vi "1_SimpleDemo_MHHisto.vi"() -> ()   [LabVIEW 2020]
uses:
  _lib/PQ/MultiHarp/MH_RefSource.ctl
  _lib/PQ/MultiHarp/MH_MeasMode.ctl
  <vilib>/Utility/error.llb/Error Cluster From Error Code.vi
  _lib/PQ/MultiHarp/MH_LibVersion_global.vi
  _lib/PQ/MultiHarp/mhlib_x86_x64_UIThread.llb/MH_DllPath_global.vi
  <vilib>/ErrorRing/Error Ring.xnode
panel:
  in  "EnableInputDeadTime":bool caption="Enable DeadTime"
  in  "InputDeadTime":i32=1000 caption="DeadTime [ps]" min=800 max=160000 step=1
  in  "Trg.Edge":i32(ring) items=["falling", "rising"]
  in  "Trg.Level":i32=-100 caption="Trg.Level [mV]" min=-1200 max=1200 step=1
  in  "Offset":i32 caption="Offset [ps]" min=-99999 max=99999 step=1
  in  "Enable":bool=TRUE
  in  "EnableSyncDeadTime":bool caption="Enable DeadTime"
  in  "SyncDeadTime":i32=1000 caption="SyncDeadTime [ps]" min=800 max=160000 step=1
  in  "SyncTrg.Edge":i32(ring) items=["falling", "rising"]
  in  "SyncTrg.Level":i32=-100 caption="SyncTrg.Level [mV]" min=-1200 max=1200 step=1
  in  "SyncOffset":i32 caption="SyncOffset [ps]" min=-99999 max=99999 step=1
  in  "SyncDivider":i32(ring)=1 items=["1"=1, "2"=2, "4"=4, "8"=8, "16"=16]
  in  "Binning":i32(ring) caption="Resolution [ps]" items=["5", "10", "20", "40", "80", "160", "320", "640", "1280", "2560", "5120", "10240", "20480", "40960", "81920", "163840", "327680", "655360", "1310720", "2621440", "5242880", "10485760", "20971520", "41943040"]
  in  "HistoLength":i32(ring)=6 caption="Histo Length" items=["1024", "2048", "4096", "8192", "16384", "32768", "65536"]
  in  "Acqu.Time":i32=10000 caption="Acqu.Time [ms]" min=1 max=360000 step=1
  in  "GlobalOffset":i32 caption="GlobalOffset [ns]" min=0 max=100000000 step=1
  in  "OverflowLevel":u32=4294967295 min=1 step=1
  in  "StopOnOverflow":bool=TRUE
  out "HistoGraph":T1(graph)={0.0, "Resolution"=0.08, "Histogram"=array8x65536[524288 elements]}
  out "CountRates":i32[](array[numeric]) caption="Count Rates [cps]"
  out "SyncRate":i32 caption="Sync Rate [cps]"
  in  "stop":bool
  out "error out":errorcluster
  # "All Channels"
  # "Sync"
  # "Acquisition"
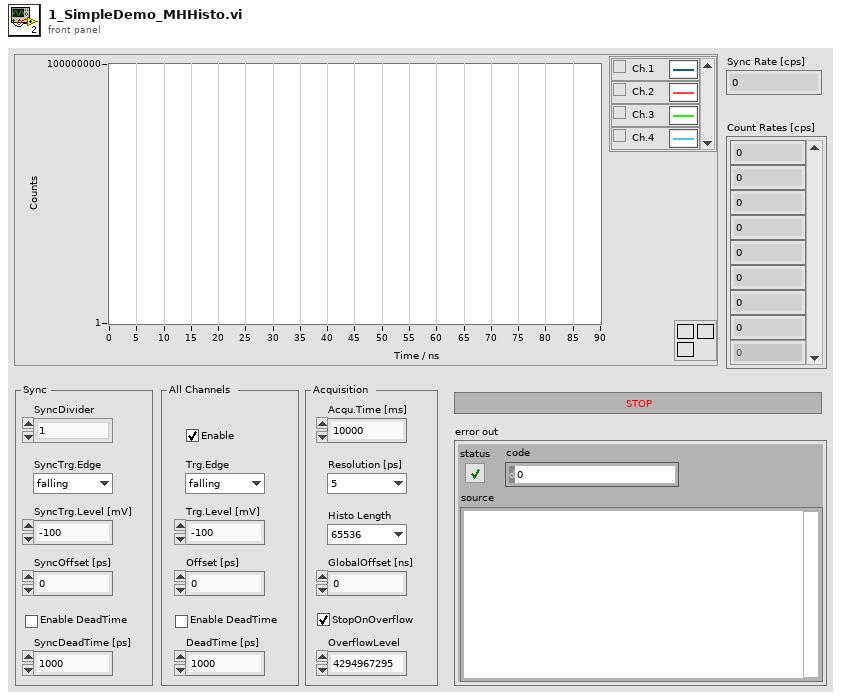
[diagram p1: front panel]
types:
  T1 = cluster{dbl, "Resolution":dbl, "Histogram":u32[][]}
  T2 = typedef "MH_MeasMode.ctl" = i32
  T3 = typedef "MH_RefSource.ctl" = enum16{"INTERNAL", "EXTERNAL_10MHZ", "WR_MASTER_GENERIC", "WR_SLAVE_GENERIC", "WR_GRANDM_GENERIC", "EXTN_GPS_PPS", "EXTN_GPS_PPS_UART", "WR_MASTER_MHARP", "WR_SLAVE_MHARP", "WR_GRANDM_MHARP"}
  T4 = typedef "MH_InitInfo.ctl" = cluster{"Library Version":string, "Serial No.":string, "Model":string, "Partnum":string, "Version":string, "features":i32, "nchannels":i32, "Base Resolution":dbl, "Bin Steps":i32}
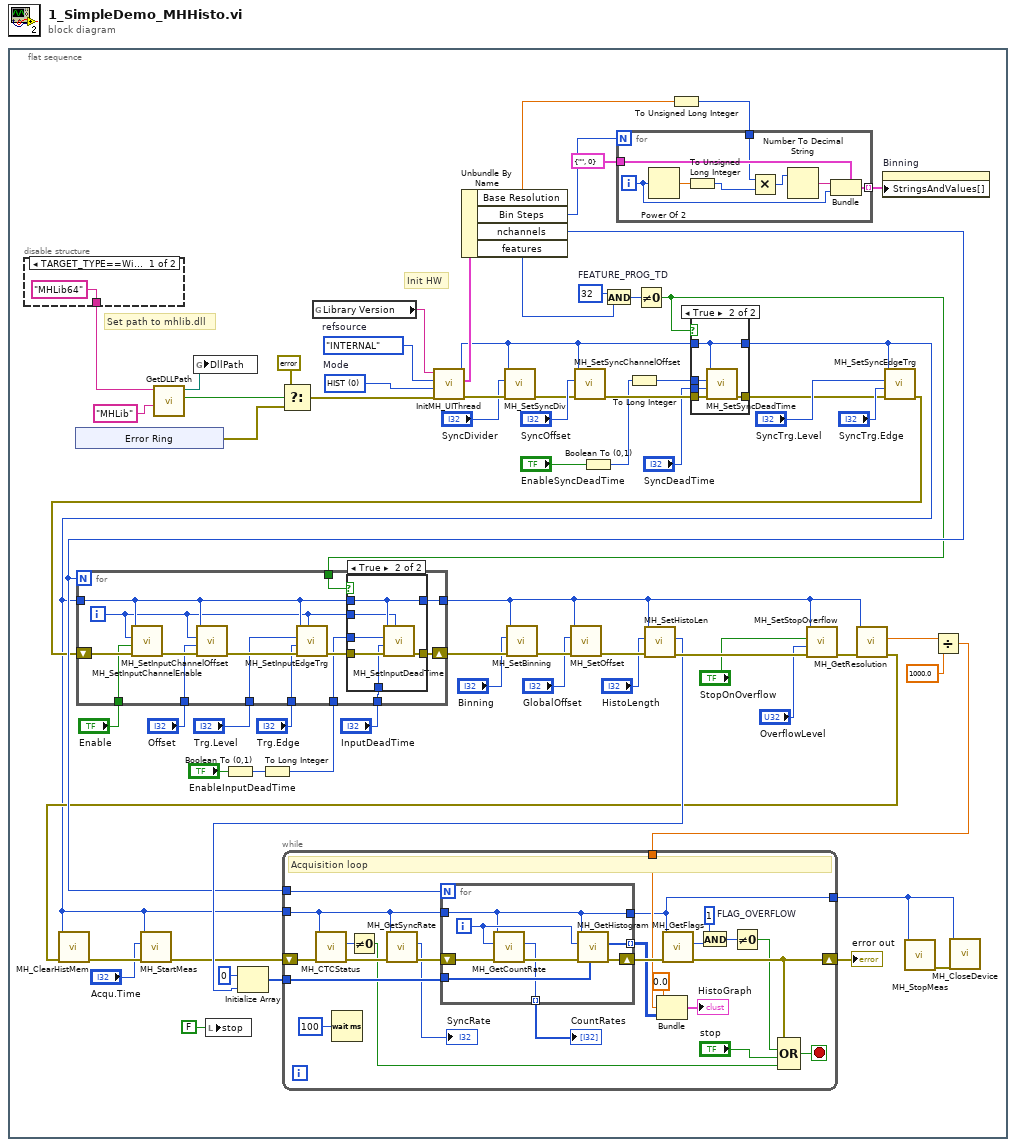
[diagram p0: block diagram]
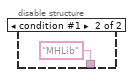
[diagram p3: hidden frame]
diagram:
  n1 = flat-sequence {
    frame #0 {
      w12 = 32  # FEATURE_PROG_TD
      w23 = T2 0 items=["HIST"=0, "T2"=2, "T3"=3]  # Mode
      w69 = MH_RefSource."INTERNAL"  # refsource
      # "Init HW"
      # "Set path to mhlib.dll"
      n2 = disable-structure shown="TARGET_TYPE==Windows, Default" {
        disable-tunnel: ["MHLib64" ("name or relative path") "MHLib" ("name or relative path")] -> w22
        frame condition #0 (active) {
        }
        frame condition #1 {
        }
      }
      n3 = xnode "Error Ring"() -> ("error out"=w68:errorcluster)
      n4 = call "GetDLLPath.vi"("DllName_32bit"="MHLib" ("name or relative path"), "DllName_64bit"=w22) -> ("file exists?"=w66:bool, "DLLPath"=w65:path)  [unwired: 8 in]
      n5 = global write "MH_DllPath_global.vi" "DllPath"(w65) -> ()
      n6 = local write "stop"(FALSE ("stop")) -> ()
      n7 = Boolean To (0,1)(Boolean="EnableInputDeadTime") -> (0, 1=w8:i16)
      n8 = To Long Integer(number=w8) -> (32bit integer=w7:i32)
      n9 = Select(t=errorcluster {"status"=FALSE, "code"=0, "source"=""} ("error IO"), s=w66, f=w68) -> (s? t:f=w63:errorcluster)
      n10 = global read "MH_LibVersion_global.vi" "Library Version"() -> (w26:string)
      n11 = call "InitMH_UIThread.vi"("error in (no error)"=w63, "Mode"=w23, "refsource"=w69, "Library Version"=w26) -> ("error out"=w58:errorcluster, "Init Info"=w60:T4, "DevIdx"=w19:i32)  [unwired: 5 in]
      n12 = Unbundle By Name(w60) -> ("Base Resolution"=w3:dbl, "Bin Steps"=w4:i32, "nchannels"=w40:i32, "features"=w14:i32)
      n13 = call "MH_SetSyncDiv.vi"("error in (no error)"=w58, "SyncDivider"="SyncDivider", "devidx"=w19) -> ("error out"=w57:errorcluster)  [unwired: 7 in, 1 out]
      n14 = call "MH_SetSyncChannelOffset.vi"("error in (no error)"=w57, "Offset"="SyncOffset", "devidx"=w19) -> ("error out"=w21:errorcluster)  [unwired: 7 in, 1 out]
      n15 = Boolean To (0,1)(Boolean="EnableSyncDeadTime") -> (0, 1=w17:i16)
      n16 = And(x=w12, y=w14) -> (x .and. y?=w13:i32)
      n17 = To Long Integer(number=w17) -> (32bit integer=w16:i32)
      n18 = Not Equal To 0?(x=w13) -> (x != 0?=w6:bool)
      n19 = To Unsigned Long Integer(number=w3) -> (unsigned 32bit integer=w2:u32)
      n20 = for {
        N: w4 -> [_]
        tunnel: cluster{"String":string, "Value":i32} {"String"="", "Value"=0} -> [w77]
        tunnel: [w71] -> w1 mode=indexing
        tunnel: w2 -> [w70]
        i -> [w76]
        n21 = Power Of 2(x=w76) -> (2^x=w75:dbl)
        n22 = To Unsigned Long Integer(number=w75) -> (unsigned 32bit integer=w74:u32)
        n23 = Multiply(x=w70, y=w74) -> (x*y=w73:u32)
        n24 = Number To Decimal String(number=w73) -> (decimal integer string=w72:string)  [unwired: 1 in]
        n25 = Bundle(cluster=w77, "String"=w72, "Value"=w76) -> (w71:cluster{"String":string, "Value":i32})
      }
      n26 = case shown="True" w6 {
        tunnel: w21 -> [w78 w84]
        tunnel: [w78 w83] -> w20
        tunnel: w19 -> [w79 w80]
        tunnel: w16 -> [_ w82]
        tunnel: "SyncDeadTime" -> [_ w81]
        tunnel: [w79 w80] -> w11
        frame False {
        }
        frame True {
          n27 = call "MH_SetSyncDeadTime.vi"("error in (no error)"=w84, "deadtime"=w81, "on"=w82, "devidx"=w80) -> ("error out"=w83:errorcluster)  [unwired: 6 in, 1 out]
        }
      }
      n28 = property on="Binning" class="Ring (strict)"("StringsAndValues[]"=w1) -> ()  [unwired: 2 in, 2 out]
      n29 = call "MH_SetSyncEdgeTrg.vi"("error in (no error)"=w20, "edge"="SyncTrg.Edge", "level"="SyncTrg.Level", "devidx"=w11) -> ("error out"=w39:errorcluster)  [unwired: 6 in, 1 out]
      n30 = for {
        N: w40 -> [_]
        shift-right: [w124] -> w59
        shift-left: w39 -> [w133]
        tunnel: w11 -> [w125]
        tunnel: [w123] -> w34
        tunnel: "Enable" -> [w130]
        tunnel: "Offset" -> [w129]
        tunnel: "Trg.Edge" -> [w128]
        tunnel: "Trg.Level" -> [w127]
        tunnel: "InputDeadTime" -> [w121]
        tunnel: w7 -> [w120]
        tunnel: w6 -> [w119]
        i -> [w122]
        n31 = call "MH_SetInputChannelEnable.vi"("error in (no error)"=w133, "enable"=w130, "channel"=w122, "devidx"=w125) -> ("error out"=w132:errorcluster)  [unwired: 6 in, 1 out]
        n32 = call "MH_SetInputChannelOffset.vi"("error in (no error)"=w132, "Offset"=w129, "channel"=w122, "devidx"=w125) -> ("error out"=w131:errorcluster)  [unwired: 6 in, 1 out]
        n33 = call "MH_SetInputEdgeTrg.vi"("channel"=w122, "error in (no error)"=w131, "edge"=w128, "level"=w127, "devidx"=w125) -> ("error out"=w126:errorcluster)  [unwired: 5 in, 1 out]
        n34 = case shown="True" w119 {
          tunnel: w126 -> [w135 w141]
          tunnel: w125 -> [w134 w139]
          tunnel: [w135 w140] -> w124
          tunnel: [w134 w139] -> w123
          tunnel: w122 -> [_ w138]
          tunnel: w121 -> [_ w137]
          tunnel: w120 -> [_ w136]
          frame False {
          }
          frame True {
            n35 = call "MH_SetInputDeadTime.vi"("channel"=w138, "error in (no error)"=w141, "deadtime"=w137, "on"=w136, "devidx"=w139) -> ("error out"=w140:errorcluster)  [unwired: 5 in, 1 out]
          }
        }
      }
      n36 = call "MH_SetBinning.vi"("error in (no error)"=w59, "Binning"="Binning", "devidx"=w34) -> ("error out"=w55:errorcluster)  [unwired: 7 in, 1 out]
      n37 = call "MH_SetOffset.vi"("error in (no error)"=w55, "Offset"="GlobalOffset", "devidx"=w34) -> ("error out"=w53:errorcluster)  [unwired: 7 in, 1 out]
      n38 = call "MH_SetHistoLen.vi"("error in (no error)"=w53, "lencode"="HistoLength", "devidx"=w34) -> ("error out"=w52:errorcluster, "actuallen"=w45:i32)  [unwired: 6 in, 1 out]
      n39 = Initialize Array(u32 0, w45) -> (w44:u32[])
      n40 = call "MH_SetStopOverflow.vi"("error in (no error)"=w52, "stopcount"="OverflowLevel", "StopOnOverflow"="StopOnOverflow", "devidx"=w34) -> ("error out"=w35:errorcluster)  [unwired: 6 in, 1 out]
      n41 = call "MH_GetResolution.vi"("error in (no error)"=w35, "devidx"=w34) -> ("error out"=w32:errorcluster, "resolution"=w33:dbl)  [unwired: 7 in, 1 out]
      n42 = call "MH_ClearHistMem.vi"("error in (no error)"=w32, "devidx"=w11) -> ("error out"=w49:errorcluster)  [unwired: 8 in, 1 out]
      n43 = call "MH_StartMeas.vi"("error in (no error)"=w49, "tacq"="Acqu.Time", "devidx"=w11) -> ("error out"=w31:errorcluster)  [unwired: 7 in, 1 out]
      n44 = Divide(x=w33, y=1000.0) -> (x/y=w41:dbl)
      n45 = while {
        shift-right: [w98] -> w47
        shift-left: w31 -> [w109]
        tunnel: w11 -> [w105]
        tunnel: w40 -> [w108]
        tunnel: w44 -> [w100]
        tunnel: w41 -> [w92]
        tunnel: [w87] -> w25
        stop <- w99 stop-if-true
        w103 = 1  # FLAG_OVERFLOW
        # "Acquisition loop"
        n46 = call "MH_CTCStatus.vi"("error in (no error)"=w109, "devidx"=w105) -> ("error out"=w107:errorcluster, "ctcstatus"=w110:i32)  [unwired: 7 in, 1 out]
        n47 = Wait (ms)(milliseconds to wait=u32 100) -> ()  [unwired: 1 out]
        n48 = Not Equal To 0?(x=w110) -> (x != 0?=w89:bool)
        n49 = call "MH_GetSyncRate.vi"("error in (no error)"=w107, "devidx"=w105) -> ("error out"=w106:errorcluster, "syncrate"=→"SyncRate":i32)  [unwired: 7 in, 1 out]
        n50 = for {
          N: w108 -> [_]
          shift-right: [w118] -> w104
          shift-left: w106 -> [w117]
          tunnel: w105 -> [w114]
          tunnel: [w114] -> w87
          tunnel: w100 -> [w113]
          tunnel: [w112] -> w95 mode=indexing
          tunnel: [w111] -> w94 mode=indexing
          i -> [w115]
          n51 = call "MH_GetCountRate.vi"("error in (no error)"=w117, "Channel"=w115, "devidx"=w114) -> ("error out"=w116:errorcluster, "rate"=w112:i32)  [unwired: 6 in, 1 out]
          n52 = call "MH_GetHistogram.vi"("Chcount"=w113, "error in (no error)"=w116, "channel"=w115, "devidx"=w114) -> ("error out"=w118:errorcluster, "Histogram"=w111:u32[])  [unwired: 5 in, 1 out]
        }
        "CountRates" <- w95
        n53 = Bundle(0.0, w92, "Histogram"=w94) -> (→"HistoGraph":cluster{dbl, dbl, "Histogram":u32[][]})  [unwired: 1 in]
        n54 = call "MH_GetFlags.vi"("error in (no error)"=w104, "devidx"=w87) -> ("error out"=w98:errorcluster, "flags"=w101:i32)  [unwired: 7 in, 1 out]
        n55 = And(x=w103, y=w101) -> (x .and. y?=w102:i32)
        n56 = Not Equal To 0?(x=w102) -> (x != 0?=w97:bool)
        n57 = Compound Arithmetic op=OR(w98, w97, "stop", w89) -> (w99:bool)
      }
      "error out" <- w47
      n58 = call "MH_StopMeas.vi"("devidx"=w25) -> ("error out"=w24:errorcluster)  [unwired: 9 in, 1 out]
      n59 = call "MH_CloseDevice.vi"("error in (no error)"=w24, "devidx"=w25) -> ()  [unwired: 8 in, 2 out]
    }
  }
